vi "HMI.vi"   [LabVIEW 2011]
doc: "This VI is called for each TeleOp packet received from the DS where the robot is not disabled. It is often used to read from the joysticks and update I/O or to update setpoints for timed control loops. It should complete and return within 20 milliseconds or it may miss DS packets."
types:
  T1 = typedef "user_data.ctl" = cluster{"Driver":cluster{"Buttons":T2, "Axes":cluster{"L-X":dbl, "L-Y":dbl, "R-X":dbl, "R-Y":dbl, "D-X":dbl, "D-Y":dbl}}, "Operator":cluster{"Buttons":T3, "Axes":cluster{"L-X":dbl, "L-Y":dbl, "Trig":dbl, "R-X":dbl, "R-Y":dbl, "D-X":dbl}}, "Kittys Kat Box":cluster{"Btn1":bool, "Btn2":bool, "Btn3":bool, "LeftKnob":dbl, "RightKnob":dbl, "SW1":bool, "SW2":bool}}
  T2 = typedef "user_buttons_dualaction.ctl" = cluster{"Btn1":bool, "Btn2":bool, "Btn3":bool, "Btn4":bool, "L1":bool, "R1":bool, "L2":bool, "R2":bool, "Face-L":bool, "Face-R":bool, "L3":bool, "R3":bool}
  T3 = typedef "user_buttons_360.ctl" = cluster{"Down":bool, "Right":bool, "Left":bool, "Up":bool, "L1":bool, "R1":bool, "Face-L":bool, "Face-R":bool, "L2":bool, "R2":bool, "Unused":bool, "Unused":bool}
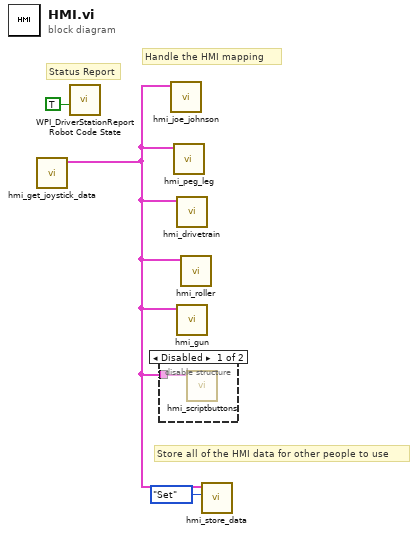
[diagram p0: block diagram]
diagram:
  # "Store all of the HMI data for other people to use"
  # "Status Report"
  # "Handle the HMI mapping"
  n1 = call "hmi_get_joystick_data.vi"() -> ("UserData"=w2:T1)  [unwired: 11 in]
  n2 = call <vilib>:"WPI_DriverStationReport Robot Code State.vi"("TeleOp"=TRUE ("Autonomous")) -> ()  [unwired: 10 in, 1 out]
  n3 = disable-structure shown="Disabled" {
    disable-tunnel: w2 -> [w4 _]
    frame Disabled {
      n4 = call "hmi_scriptbuttons.vi"("UserData"=w4) -> ()  [unwired: 11 in]
    }
    frame Enabled {
    }
  }
  n5 = call "hmi_joe_johnson.vi"("UserData"=w2) -> ()  [unwired: 11 in]
  n6 = call "hmi_peg_leg.vi"("UserData"=w2) -> ()  [unwired: 11 in]
  n7 = call "hmi_drivetrain.vi"("UserData"=w2) -> ()  [unwired: 11 in]
  n8 = call "hmi_gun.vi"("UserData"=w2) -> ()  [unwired: 11 in]
  n9 = call "hmi_roller.vi"("UserData"=w2) -> ()  [unwired: 11 in]
  n10 = call "hmi_store_data.vi"("data_store_mode"=enum16{"Set", "Get"}."Set", "UserData"=w2) -> ()  [unwired: 9 in, 1 out]
